vi "Read Analogue.vi"(8 "error in (no error)":errorcluster, 11 "APS 7050":refnum<class "APS 7050.lvclass">) -> (0 "error out":errorcluster, 2 "Waveforms":waveform(dbl)[](array[waveform]), 3 "APS 7050 out":refnum<class "APS 7050.lvclass">)   [LabVIEW 2025, in "Power Supply.lvlib" / "APS 7050.lvclass"]
uses:
  APS 7050.lvclass
  C:/Users/Public/Documents/Sandia National Labs/TSS Plugin/Abstract Engine.lvlibp/Abstract Instrument/Abstract Instrument.lvclass
  APS 7050.lvclass/APS 7050.ctl
  <instrlib>/APS-7000 Series/APS-7000 Series.lvlib
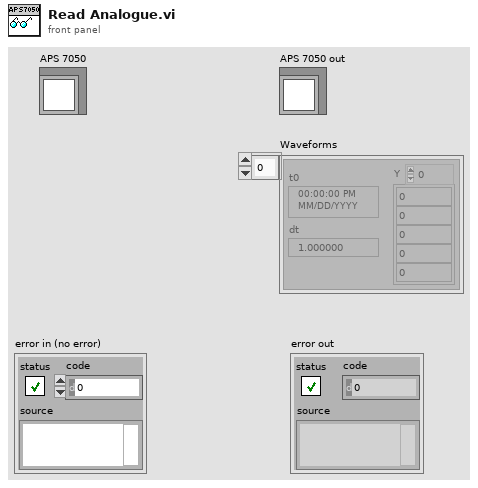
[diagram p1: front panel]
types:
  T1 = typedef "Abstract Engine.lvlibp/Abstract Instrument.lvclass/Channel.ctl" = cluster{"Alias":string, "DataType":enum16{"Anaolg Input", "Waveform"}, "Unit":enum16{"---", "V", "A", "Ohm", "Hz", "uF", "degC", "deg"}, "Upper limit":dbl, "Lower limit":dbl, "Measurement":variant}
  T2 = cluster{"Vmeas? (Vrms)":dbl, "Imeas? (Arms)":dbl}
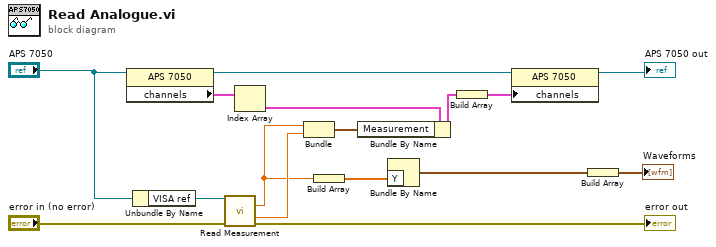
[diagram p0: block diagram]
diagram:
  n1 = property class="APS 7050"(reference="APS 7050") -> (reference out=w11:refnum<class "APS 7050.lvclass">, "channels"=w10:T1[])  [unwired: 1 in, 1 out]
  n2 = Unbundle By Name("APS 7050") -> ("VISA ref"=w14:refnum<visa-resource-name>)
  n3 = call <instrlib>:"Read Measurement.vi"("VISA in"=w14, "error in"="error in (no error)") -> ("Vmeas? (Vrms)"=w4:dbl, "Imeas? (Arms)"=w8:dbl, "error out"=→"error out":errorcluster)  [unwired: 3 in, 8 out]
  n4 = Index Array(array=w10) -> (element=w5:T1)  [unwired: 1 in]
  n5 = Bundle("Vmeas? (Vrms)"=w4, "Imeas? (Arms)"=w8) -> (w7:T2)  [unwired: 1 in]
  n6 = Build Array(w4) -> (w3:dbl[])
  n7 = Bundle By Name(cluster=w5, "Measurement"=w7) -> (w9:T1)
  n8 = Bundle By Name("Y"=w3) -> (w2:waveform(dbl))  [unwired: 1 in]
  n9 = Build Array(w9) -> (w6:T1[])
  n10 = property class="APS 7050"(reference=w11, "channels"=w6) -> (reference out=→"APS 7050 out":refnum<class "APS 7050.lvclass">)  [unwired: 1 in, 1 out]
  n11 = Build Array(w2) -> (→"Waveforms":waveform(dbl)[])
